vi "Expand.vi"(8 "error in (no error)":errorcluster, 10 "IB_Tree.lvclass":refnum<class "IB_Tree.lvclass">, 11 "IB_TreeRootItem in":refnum<class "IB_Tree_Item_Proj_BuildSpecs.lvclass">) -> (0 "error out":errorcluster, 2 "first expansion?":bool, 3 "IB_TreeRootItem out":refnum<class "IB_Tree_Item_Proj_BuildSpecs.lvclass">)   [LabVIEW 2020, in "IB_Tree_Item_Proj_BuildSpecs.lvclass"]
uses:
  <vilib>/AppBuilder/IB_Classes/Tree_Item_Proj_BuildSpecs/IB_Tree_Item_Proj_BuildSpecs.lvclass
  <vilib>/AppBuilder/IB_Classes/Tree_Item_Proj_BuildSpecs/IB_Tree_Item_Proj_BuildSpecs.lvclass/IB_Tree_Item_Proj_BuildSpecs.ctl
  <vilib>/AppBuilder/IB_Classes/Tree_Source/IB_Tree_Source.lvclass
  <resource>/Framework/Providers/Builds/Installer/controls/IB_sTypeDef_BuildTypes.ctl
  <vilib>/AppBuilder/IB_Classes/Tree_Item_Proj_Build/IB_Tree_Item_Proj_Build.lvclass
  <vilib>/AppBuilder/IB_Classes/Tree_Item/IB_Tree_Item.lvclass
  <vilib>/AppBuilder/IB_Classes/Tree_Item_Proj/IB_Tree_Item_Proj.lvclass
  <vilib>/AppBuilder/IB_Classes/Tree_Item_Proj_EXE/IB_Tree_Item_Proj_EXE.lvclass
  <vilib>/AppBuilder/IB_Classes/Tree_Item_Proj_DLL/IB_Tree_Item_Proj_DLL.lvclass
  <vilib>/AppBuilder/IB_Classes/Tree_Item_Proj_SDIST/IB_Tree_Item_Proj_SDIST.lvclass
  <vilib>/AppBuilder/IB_Classes/Tree_Item_Proj_RestfulWS/IB_Tree_Item_Proj_RestfulWS.lvclass
  <vilib>/AppBuilder/IB_Classes/Tree_Item_Proj_NET/IB_Tree_Item_Proj_NET.lvclass
  <vilib>/AppBuilder/IB_Classes/Tree_Item_Proj_PackedLib/IB_Tree_Item_Proj_PackedLib.lvclass
  <vilib>/AppBuilder/IB_Classes/Tree_Item_Proj_Container/IB_Tree_Item_Proj_Container.lvclass
  e:/builds/penguin/labview/branches/2020/dev/dist/vi.lib/AppBuilder/IB_Classes/Tree_Item_Proj_Container/IB_Tree_Item_Proj_Container.lvclass
  e:/builds/penguin/labview/branches/2020/dev/dist/vi.lib/AppBuilder/IB_Classes/Tree_Item_Proj/IB_Tree_Item_Proj.lvclass
  e:/builds/penguin/labview/branches/2020/dev/dist/vi.lib/AppBuilder/IB_Classes/Tree_Item/IB_Tree_Item.lvclass
  e:/builds/penguin/labview/branches/2020/dev/dist/vi.lib/AppBuilder/IB_Classes/Tree_Item_Proj_Build/IB_Tree_Item_Proj_Build.lvclass
  e:/builds/penguin/labview/branches/2020/dev/dist/vi.lib/AppBuilder/IB_Classes/Tree_Item_Proj_BuildSpecs/IB_Tree_Item_Proj_BuildSpecs.lvclass
  e:/builds/penguin/labview/branches/2020/dev/dist/vi.lib/AppBuilder/IB_Classes/Tree_Item_Proj_EXE/IB_Tree_Item_Proj_EXE.lvclass
  e:/builds/penguin/labview/branches/2020/dev/dist/vi.lib/AppBuilder/IB_Classes/Tree_Item_Proj_DLL/IB_Tree_Item_Proj_DLL.lvclass
  e:/builds/penguin/labview/branches/2020/dev/dist/vi.lib/AppBuilder/IB_Classes/Tree_Item_Proj_SDIST/IB_Tree_Item_Proj_SDIST.lvclass
  e:/builds/penguin/labview/branches/2020/dev/dist/vi.lib/AppBuilder/IB_Classes/Tree_Item_Proj_RestfulWS/IB_Tree_Item_Proj_RestfulWS.lvclass
  e:/builds/penguin/labview/branches/2020/dev/dist/vi.lib/AppBuilder/IB_Classes/Tree_Item_Proj_NET/IB_Tree_Item_Proj_NET.lvclass
  e:/builds/penguin/labview/branches/2020/dev/dist/vi.lib/AppBuilder/IB_Classes/Tree_Item_Proj_PackedLib/IB_Tree_Item_Proj_PackedLib.lvclass
  e:/builds/penguin/labview/branches/2020/dev/dist/vi.lib/AppBuilder/IB_Classes/Tree/IB_Tree.lvclass
  e:/builds/penguin/labview/branches/2020/dev/dist/vi.lib/AppBuilder/IB_Classes/Tree_Source/IB_Tree_Source.lvclass
  <vilib>/AppBuilder/IB_Classes/Tree/IB_Tree.lvclass
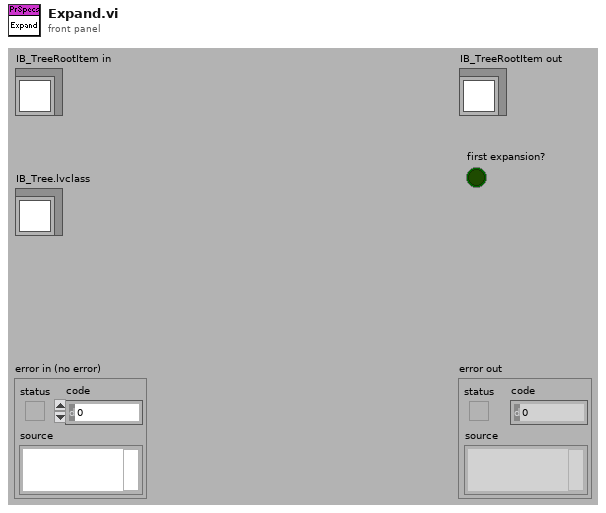
[diagram p1: front panel]
types:
  T1 = typedef "IB_sTypeDef_BuildTypes.ctl" = enum16{"Invalid", "EXE", "DLL", "Source Distribution", "RESTful WS", ".NET", "Packed Library"}
  T2 = typedef "IB_Tree_Item.ctl" = cluster{"symbol index":i32, "child tag":string, "parentTag":string, "left cell name":string}
  T3 = typedef "IB_Tree_Source.ctl" = cluster{"buildObject":T4}
  T4 = typedef "ItemRef.ctl" = u64
  T5 = typedef "IB_Tree_Item_Proj.ctl" = cluster{"itemID":string, "path":path}
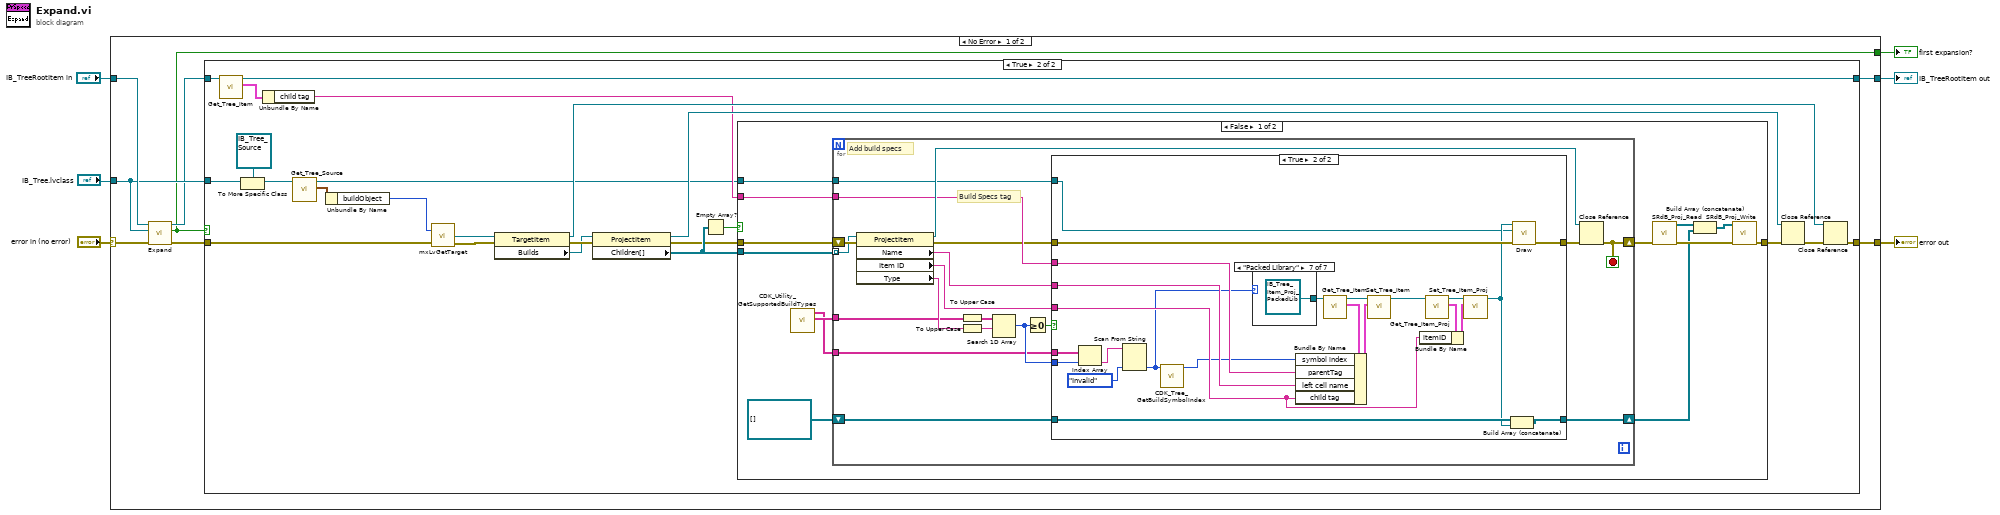
[diagram p0: block diagram]
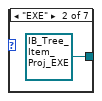
[diagram p5: hidden frame]
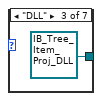
[diagram p6: hidden frame]
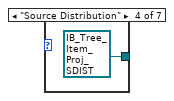
[diagram p7: hidden frame]
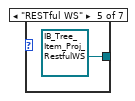
[diagram p8: hidden frame]
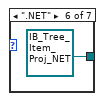
[diagram p9: hidden frame]
diagram:
  n1 = case shown="No Error" "error in (no error)" {
    selector: "error in (no error)" -> [w13 w105]
    tunnel: [w11 w105] -> w6
    tunnel: [w7 _] -> w5
    tunnel: [w8 w104] -> w4
    tunnel: "IB_Tree.lvclass" -> [w10 _]
    tunnel: "IB_TreeRootItem in" -> [w14 w104]
    frame No Error {
      n2 = call-parent "Expand.vi"("error in (no error)"=w13, "IB_Tree.lvclass"=w10, "IB_TreeRootItem in"=w14) -> ("error out"=w12:errorcluster, "first expansion?"=w7:bool, "IB_TreeRootItem out"=w9:refnum<class "IB_Tree_Item_Proj_BuildSpecs.lvclass">)  [unwired: 6 out]
      n3 = case shown="True" w7 {
        tunnel: w12 -> [w16 w18]
        tunnel: [w16 w27] -> w11
        tunnel: w10 -> [_ w22]
        tunnel: w9 -> [w15 w26]
        tunnel: [w15 w25] -> w8
        frame False {
        }
        frame True {
          n4 = call <vilib>:"Get_Tree_Item.vi"("IB_TreeItem in"=w26) -> ("data"=w24:T2, "IB_TreeItem out"=w25:refnum<class "IB_Tree_Item_Proj_BuildSpecs.lvclass">)  [unwired: 1 in, 8 out]
          n5 = To More Specific Class(target class=refnum<class "IB_Tree_Source.lvclass"> refnum ("IB_SourceTree.lvclass"), reference=w22) -> (specific class reference=w30:refnum<class "IB_Tree_Source.lvclass">)  [unwired: 1 in, 1 out]
          n6 = Unbundle By Name(w24) -> ("child tag"=w23:string)
          n7 = call <vilib>:"Get_Tree_Source.vi"("IB_SourceTree in"=w30) -> ("data"=w28:T3, "IB_SourceTree out"=w21:refnum<class "IB_Tree_Source.lvclass">)  [unwired: 1 in, 8 out]
          n8 = Unbundle By Name(w28) -> ("buildObject"=w20:T4)
          n9 = call <resource>:"mxLvGetTarget.vi"("Item"=w20, "error in"=w18) -> ("Target"=w19:refnum<vi>, "error out"=w17:errorcluster)  [unwired: 1 out]
          n10 = property class="TargetItem"(reference=w19, error in=w17) -> (reference out=w39:refnum<vi>, error out=w32:errorcluster, "Builds"=w31:refnum<vi>)
          n11 = property class="ProjectItem"(reference=w31, error in=w32) -> (reference out=w38:refnum<vi>, error out=w34:errorcluster, "Children[]"=w35:refnum<vi>[])
          n12 = Empty Array?(array=w35) -> (empty?=w33:bool)
          n13 = case shown="False" w33 {
            tunnel: w34 -> [w52 w103]
            tunnel: w35 -> [w51 _]
            tunnel: [w43 w103] -> w37
            tunnel: w23 -> [w50 _]
            tunnel: w21 -> [w48 _]
            frame False {
              n14 = call <resource>:"CDK_Utility_GetSupportedBuildTypes.vi"() -> ("type GUIDs"=w41:string[], "type strings"=w40:string[])  [unwired: 1 in, 9 out]
              n15 = for {
                tunnel: w51 -> [w68] mode=indexing
                shift-right: [w61] -> w44
                shift-left: w52 -> [w69]
                tunnel: w41 -> [w53]
                tunnel: w50 -> [w59]
                shift-right: [w56] -> w42
                shift-left: refnum<class "IB_Tree_Item_Proj_Build.lvclass">[] [] -> [w57]
                tunnel: w48 -> [w55]
                tunnel: w40 -> [w54]
                stop <- w61 stop-if-true
                # "Build Specs tag"
                # "Add build specs"
                n16 = property class="ProjectItem"(reference=w68, error in=w69) -> (reference out=w62:refnum<vi>, error out=w58:errorcluster, "Name"=w70:string, "Item ID"=w71:string, "Type"=w64:string)
                n17 = To Upper Case(1:w53) -> (0:w66:string[])
                n18 = To Upper Case(1:w64) -> (0:w67:string)
                n19 = Search 1D Array(1D array=w66, element=w67) -> (index of element=w60:i32)  [unwired: 1 out]
                n20 = Greater Or Equal To 0?(x=w60) -> (x >= 0?=w65:bool)
                n21 = case shown="True" w65 {
                  tunnel: w71 -> [_ w80]
                  tunnel: w59 -> [_ w86]
                  tunnel: w70 -> [_ w85]
                  tunnel: w58 -> [w73 w78]
                  tunnel: [w73 w77] -> w63
                  tunnel: w54 -> [_ w96]
                  tunnel: w60 -> [_ w95]
                  tunnel: w57 -> [w72 w88]
                  tunnel: [w72 w87] -> w56
                  tunnel: w55 -> [_ w75]
                  frame False {
                  }
                  frame True {
                    n22 = Index Array(array=w96, index=w95) -> (element=w93:string)
                    n23 = Scan From String(input string=w93, default 1=IB_sTypeDef_BuildTypes."Invalid" ("buildTypes")) -> (output 1=w74:T1)  [unwired: 3 in, 3 out]
                    n24 = call <resource>:"CDK_Tree_GetBuildSymbolIndex.vi"("buildType"=w74) -> ("symbol index"=w79:i32)  [unwired: 1 in, 9 out]
                    n25 = case shown="\"Packed Library\"" w74 {
                      tunnel: [_ refnum<class "IB_Tree_Item_Proj_EXE.lvclass"> refnum ("IB_Tree_Item_Proj_EXE.lvclass") refnum<class "IB_Tree_Item_Proj_DLL.lvclass"> refnum ("IB_Tree_Item_Proj_DLL.lvclass") refnum<class "IB_Tree_Item_Proj_SDIST.lvclass"> refnum ("IB_Tree_Item_Proj_SDIST.lvclass") refnum<class "IB_Tree_Item_Proj_RestfulWS.lvclass"> refnum ("IB_Tree_Item_Proj_RestfulWS.lvclass") refnum<class "IB_Tree_Item_Proj_NET.lvclass"> refnum ("IB_Tree_Item_Proj_NET.lvclass") refnum<class "IB_Tree_Item_Proj_PackedLib.lvclass"> refnum ("IB_Tree_Item_Proj_PackedLib.lvclass")] -> w89
                      frame Default {
                      }
                      frame "EXE" {
                      }
                      frame "DLL" {
                      }
                      frame "Source Distribution" {
                      }
                      frame "RESTful WS" {
                      }
                      frame ".NET" {
                      }
                      frame "Packed Library" {
                      }
                    }
                    n26 = call <vilib>:"Get_Tree_Item.vi"("IB_TreeItem in"=w89) -> ("data"=w90:T2, "IB_TreeItem out"=w92:refnum<class "IB_Tree_Item_Proj_Build.lvclass">)  [unwired: 1 in, 8 out]
                    n27 = Bundle By Name(cluster=w90, "symbol index"=w79, "parentTag"=w86, "left cell name"=w85, "child tag"=w80) -> (w91:T2)
                    n28 = call <vilib>:"Set_Tree_Item.vi"("data"=w91, "IB_TreeItem in"=w92) -> ("IB_TreeItem out"=w81:refnum<class "IB_Tree_Item_Proj_Build.lvclass">)  [unwired: 1 in, 8 out]
                    n29 = call <vilib>:"Get_Tree_Item_Proj.vi"("IB_TreeProjectItem in"=w81) -> ("data"=w83:T5, "IB_TreeProjectItem out"=w84:refnum<class "IB_Tree_Item_Proj_Build.lvclass">)  [unwired: 1 in, 8 out]
                    n30 = Bundle By Name(cluster=w83, "itemID"=w80) -> (w82:T5)
                    n31 = call <vilib>:"Set_Tree_Item_Proj.vi"("data"=w82, "IB_TreeProjectItem in"=w84) -> ("IB_TreeProjectItem out"=w76:refnum<class "IB_Tree_Item_Proj_Build.lvclass">)  [unwired: 1 in, 8 out]
                    n32 = Build Array (concatenate)(w88, w76) -> (w87:refnum<class "IB_Tree_Item_Proj_Build.lvclass">[])
                    n33 = call-dynamic "Draw.vi"("error in (no error)"=w78, "IB_Tree"=w75, "IB_TreeProjContainer in"=w76) -> ("error out"=w77:errorcluster)  [unwired: 1 in, 7 out]
                  }
                }
                n34 = Close Reference(reference=w62, error in (no error)=w63) -> (error out=w61:errorcluster)
              }
              n35 = call <resource>:"SRdB_Proj_Read.vi"("error in (no error)"=w44) -> ("error out"=w45:errorcluster, "Proj Items"=w47:refnum<class "IB_Tree_Item_Proj.lvclass">[])  [unwired: 9 out]
              n36 = Build Array (concatenate)(w47, w42) -> (w46:refnum<class "IB_Tree_Item_Proj.lvclass">[])
              n37 = call <resource>:"SRdB_Proj_Write.vi"("error in (no error)"=w45, "Proj Items"=w46) -> ("error out"=w43:errorcluster)  [unwired: 9 out]
            }
            frame True {
            }
          }
          n38 = Close Reference(reference=w38, error in (no error)=w37) -> (error out=w36:errorcluster)
          n39 = Close Reference(reference=w39, error in (no error)=w36) -> (error out=w27:errorcluster)
        }
      }
    }
    frame Error {
    }
  }
  "error out" <- w6
  "IB_TreeRootItem out" <- w4
  "first expansion?" <- w5
